vi "Append Path to Root if Relative__ogtk.vi"   [LabVIEW 2018]
doc: "Ouputs \"Absolute or Relative Path\". If \"Absolute or Relative Path\" is relative it is appended to \"Root Path\". If \"Absolute or Relative Path\" is absolute it is passed straight through."
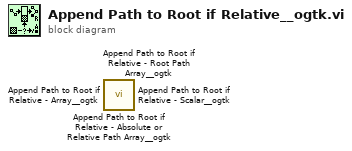
[diagram p0: block diagram]
diagram:
  n1 = call <userlib>:"Append Path to Root if Relative - Absolute or Relative Path Array__ogtk.vi"() -> ()  [unwired: 2 in, 1 out]
  n2 = call <userlib>:"Append Path to Root if Relative - Root Path Array__ogtk.vi"() -> ()  [unwired: 2 in, 1 out]
  n3 = call <userlib>:"Append Path to Root if Relative - Array__ogtk.vi"() -> ()  [unwired: 2 in, 1 out]
  n4 = call <userlib>:"Append Path to Root if Relative - Scalar__ogtk.vi"() -> ()  [unwired: 2 in, 1 out]
